vi "Get Value.vi"(9 "Label":string, 10 "Cluster":T1) -> (2 "Val":i32)   [LabVIEW 2021, in "Rule.lvclass"]
uses:
  Rule.lvclass
  Rule.lvclass/Rule.ctl
  xmas.ctl
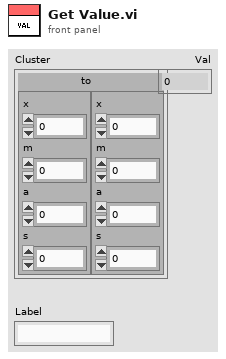
[diagram p1: front panel]
types:
  T1 = typedef "xmas.ctl" = cluster{"from":cluster{"x":u64, "m":u64, "a":u64, "s":u64}, "to":cluster{"x":u64, "m":u64, "a":u64, "s":u64}}
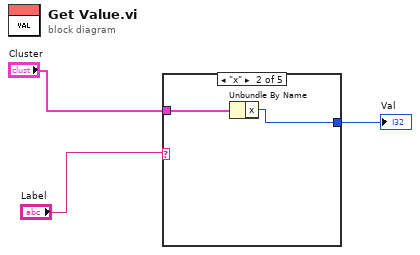
[diagram p0: block diagram]
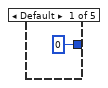
[diagram p2: hidden frame]
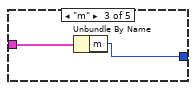
[diagram p3: hidden frame]
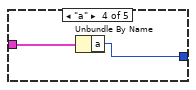
[diagram p4: hidden frame]
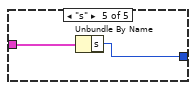
[diagram p5: hidden frame]
diagram:
  n1 = case shown="\"x\"" "Label" {
    tunnel: "Cluster" -> [_ w6 w8 w10 w12]
    tunnel: [0 ("s") w5 w7 w9 w11] -> w1
    frame Default {
    }
    frame "x" {
      n2 = Unbundle By Name(w6) -> ("x"=w5:i32)
    }
    frame "m" {
      n3 = Unbundle By Name(w8) -> ("m"=w7:i32)
    }
    frame "a" {
      n4 = Unbundle By Name(w10) -> ("a"=w9:i32)
    }
    frame "s" {
      n5 = Unbundle By Name(w12) -> ("s"=w11:i32)
    }
  }
  "Val" <- w1
